vi "UI.vi"() -> ()   [LabVIEW 2014]
uses:
  Tasks.ctl
panel:
  in  "Log File Path":path=path "C:/Users/Dany/Documents/GitHub/Health Tracker/Pulse-Oximetry/data.tdms"
  out "Waveform Chart":dbl[][](graph)
  out "Stops":bool
  in  "myRIO IP":string="172.22.11.2"
  in  "Off":bool
  in  "LED1":bool
  in  "LED2":bool
  in  "Stop Button":bool
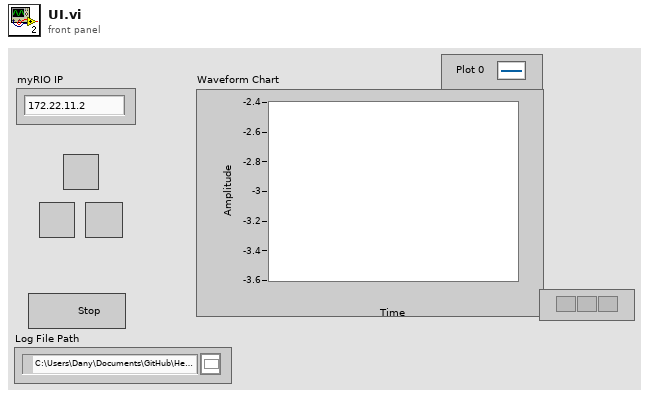
[diagram p1: front panel]
types:
  T1 = enum16{"open", "open or create", "create or replace", "create", "open (read-only)"}
  T2 = typedef "Tasks.ctl" = enum16{"Stop", "LEDs Off", "LED1 On", "LED2 On"}
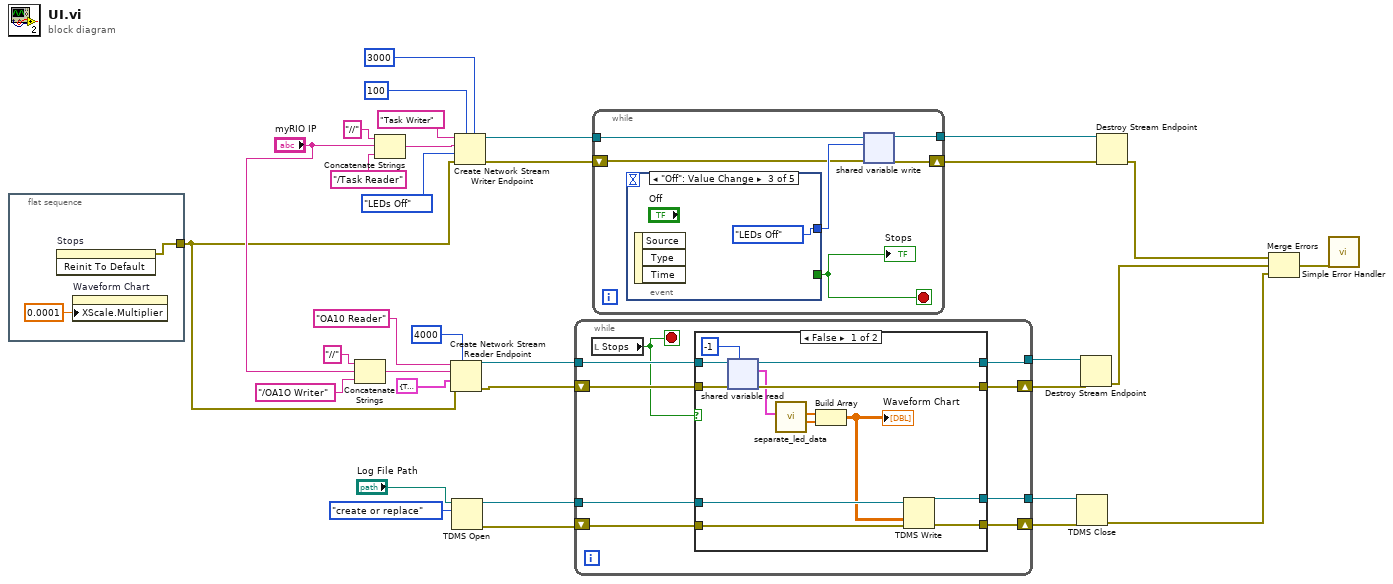
[diagram p0: block diagram]
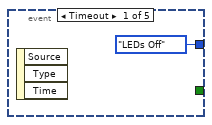
[diagram p3: hidden frame]
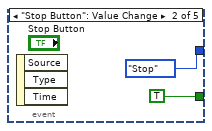
[diagram p4: hidden frame]
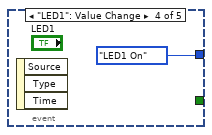
[diagram p5: hidden frame]
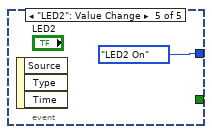
[diagram p6: hidden frame]
diagram:
  n1 = flat-sequence {
    tunnel: [w35] -> w5
    frame #0 {
      n2 = invoke on="Stops" class="Bool (strict)" method="Reinit To Default"() -> (error out=w35:errorcluster)  [unwired: 3 in, 2 out]
      n3 = property on="Waveform Chart" class="WFChart (strict)"("XScale.Multiplier"=0.0001 ("X Scale.Offset and Multiplier:Multiplier")) -> ()  [unwired: 2 in, 2 out]
    }
  }
  n4 = Concatenate Strings("//" ("string"), "myRIO IP", "/OA1O Writer" ("string")) -> (w17:string)
  n5 = Concatenate Strings("//" ("string"), "myRIO IP", "/Task Reader" ("string")) -> (w31:string)
  n6 = Create Network Stream Reader Endpoint(7:4000 ("reader buffer size"), 8:w5, 9:cluster{"LED1?":bool, "Data":dbl} {"LED1?"=TRUE, "Data"=0.0}, 10:w17, 11:"OA10 Reader" ("reader name")) -> (0:w14:errorcluster, 3:w15:refnum<k21>)  [unwired: 2 in]
  n7 = TDMS Open(10:T1."create or replace" ("operation (0:open)"), 11:"Log File Path") -> (0:w24:errorcluster, 3:w25:refnum<k34>)  [unwired: 5 in]
  n8 = Create Network Stream Writer Endpoint(5:3000 ("timeout in ms (-1)"), 7:100 ("writer buffer size"), 8:w5, 9:Tasks."LEDs Off" ("Tasks"), 10:w31, 11:"Task Writer" ("writer name")) -> (0:w26:errorcluster, 3:w2:refnum<k21>)  [unwired: 1 in]
  n9 = while {
    tunnel: w25 -> [w44]
    tunnel: w15 -> [w42]
    tunnel: [w40] -> w13
    shift-right: [w39] -> w12
    shift-left: w14 -> [w41]
    shift-right: [w38] -> w11
    shift-left: w24 -> [w43]
    tunnel: [w37] -> w10
    stop <- w36 stop-if-true
    n10 = local read "Stops"() -> (w36:bool)
    n11 = case shown="False" w36 {
      tunnel: w44 -> [w57 w59]
      tunnel: w43 -> [w56 w58]
      tunnel: w42 -> [w55 w61]
      tunnel: w41 -> [w54 w60]
      tunnel: [w53 w61] -> w40
      tunnel: [w52 w60] -> w39
      tunnel: [w51 w58] -> w38
      tunnel: [w50 w59] -> w37
      frame False {
        n12 = shared-variable-read(w55, w54, -1 ("# elements")) -> (w53:refnum<k21>, w52:errorcluster, w48:cluster{"LED1?":bool, "Data":dbl}[])  [unwired: 1 in, 1 out]
        n13 = call "separate_led_data.vi"("Data from Stream"=w48) -> ("LED2"=w46:dbl[], "LED1"=w47:dbl[])  [unwired: 9 in]
        n14 = Build Array(w47, w46) -> (w45:dbl[][])
        "Waveform Chart" <- w45
        n15 = TDMS Write(0:w57, 9:w45, 11:w56) -> (4:w50:refnum<k34>, 15:w51:errorcluster)  [unwired: 3 in, 2 out]
      }
      frame True {
      }
    }
  }
  n16 = while {
    tunnel: w2 -> [w62]
    tunnel: [w65] -> w3
    shift-right: [w64] -> w4
    shift-left: w26 -> [w66]
    stop <- w63 stop-if-true
    n17 = event shown="[2] \"Off\": Value Change" {
      selector: _ -> [_ _ _ _ _]
      dyn-events: _ -> [_ _ _ _ _]
      timeout: _ -> [_ _ _ _ _]
      tunnel: [Tasks."LEDs Off" ("Tasks") Tasks."Stop" ("Tasks") Tasks."LEDs Off" ("Tasks") Tasks."LED1 On" ("Tasks") Tasks."LED2 On" ("Tasks")] -> w67
      tunnel: [_ TRUE _ _ _] -> w63
      event Timeout {
        n18 = event-data() -> ()  [unwired: 1 in, 3 out]
      }
      event "Stop Button": Value Change {
        n19 = event-data() -> ()  [unwired: 1 in, 3 out]
      }
      event "Off": Value Change {
        n20 = event-data() -> ()  [unwired: 1 in, 3 out]
      }
      event "LED1": Value Change {
        n21 = event-data() -> ()  [unwired: 1 in, 3 out]
      }
      event "LED2": Value Change {
        n22 = event-data() -> ()  [unwired: 1 in, 3 out]
      }
    }
    "Stops" <- w63
    n23 = shared-variable-write(w62, w66, w67) -> (w65:refnum<k21>, w64:errorcluster)  [unwired: 1 in, 1 out]
  }
  n24 = TDMS Close(8:w11, 11:w10) -> (0:w7:errorcluster)  [unwired: 1 out]
  n25 = Destroy Stream Endpoint(8:w12, 11:w13) -> (0:w8:errorcluster)
  n26 = Destroy Stream Endpoint(8:w4, 11:w3) -> (0:w9:errorcluster)
  n27 = Merge Errors(w9, w8, w7) -> (w6:errorcluster)
  n28 = call <vilib>:"Simple Error Handler.vi"("error in (no error)"=w6) -> ()  [unwired: 4 in, 5 out]
